vi "Initialize.vi"(8 "error in":errorcluster, 11 "Plugin in":refnum<class "StreamReader.lvclass">) -> (0 "error out":errorcluster, 3 "Plugin out":refnum<class "StreamReader.lvclass">)   [LabVIEW 2024, in "StreamReader.lvlib" / "StreamReader.lvclass"]
uses:
  StreamReader.lvclass
  C:/Program Files/National Instruments/LabVIEW 2024/vi.lib/FlexLogger/SDK/PluginSDK.lvlibp/PEFClasses/SDK/Plugin/Plugin.lvclass
  StreamReader Parameters.ctl
  <vilib>/FlexLogger/SDK/PluginSDK.lvlibp/PEFClasses/SDK/Processing Element/Timing Parameters.ctl
  <vilib>/FlexLogger/SDK/PluginSDK.lvlibp/PEFClasses/SDK/Processing Element/Timing Method.ctl
  StreamReader.lvclass/StreamReader.ctl
  StreamReader Strings.vi
  <vilib>/FlexLogger/SDK/PluginSDK.lvlibp/PEFClasses/SDK/Plugin/ParameterAccess/Write String.vi
  <vilib>/FlexLogger/SDK/PluginSDK.lvlibp/PEFClasses/SDK/Plugin/ParameterAccess/Write I32.vi
  <vilib>/FlexLogger/SDK/PluginSDK.lvlibp/PEFClasses/SDK/Plugin/Plugin.lvclass
  C:/Program Files/National Instruments/LabVIEW 2024/vi.lib/FlexLogger/SDK/PluginSDK.lvlibp/PEFClasses/SDK/Processing Element/Processing Element.lvclass
  C:/dev/niflexlogger-plugins/plugins/StreamReader/source/StreamReader/StreamReader.lvclass
  <vilib>/FlexLogger/SDK/PluginSDK.lvlibp/PEFClasses/SDK/Processing Element/Processing Element.lvclass
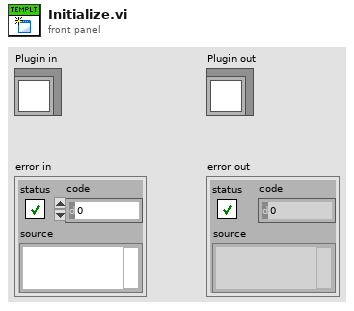
[diagram p1: front panel]
types:
  T1 = typedef "PluginSDK.lvlibp/Processing Element.lvclass/Timing Parameters.ctl" = cluster{"Timing Method":T2, "Timing Period (ms)":i32}
  T2 = typedef "PluginSDK.lvlibp/Processing Element.lvclass/Timing Method.ctl" = enum16{"Periodic", "Immediate", "On Data Ready", "Triggered"}
  T3 = typedef "StreamReader.lvlib/StreamReader.lvclass/StreamReader Parameters.ctl" = cluster{"Reader URL":string, "Writer URL":string, "Buffer Size":i32, "Reader endpoint":refnum<k21>, "Channel Names":string[]}
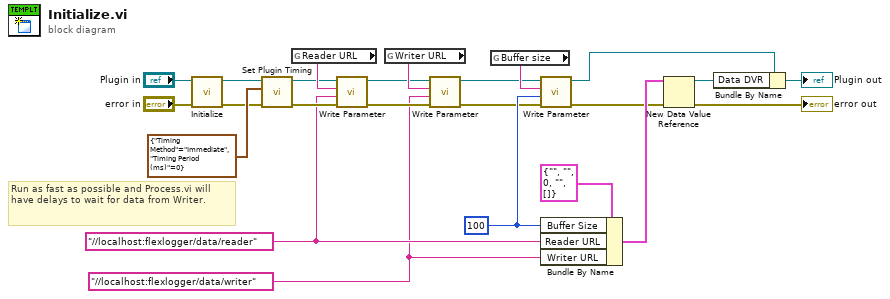
[diagram p0: block diagram]
diagram:
  w2 = "//localhost:flexlogger/data/reader" ("Value")
  w12 = 100 ("Value")
  w1 = "//localhost:flexlogger/data/writer" ("Value")
  # "Run as fast as possible and Process.vi will have delays to wait for data from Writer."
  n1 = call-parent "Initialize.vi"("error in (no error)"="error in", "Plugin in"="Plugin in") -> ("error out"=w6:errorcluster, "Plugin out"=w8:refnum<class "StreamReader.lvclass">)  [unwired: 8 in]
  n2 = call <vilib>:"Set Plugin Timing.vi"("error in (no error)"=w6, "Timing Parameters"=T1 {"Timing Method"=enum."Immediate", "Timing Period (ms)"=0}, "Plugin in"=w8) -> ("error out"=w5:errorcluster, "Plugin out"=w7:refnum<class "StreamReader.lvclass">)  [unwired: 7 in]
  n3 = global read "StreamReader Strings.vi" "Reader URL"() -> (w20:string)
  n4 = call-poly <vilib>:"Write Parameter.vi"("error in (no error)"=w5, "Value"=w2, "Name"=w20, "Plugin in"=w7) -> ("error out"=w18:errorcluster, "Plugin out"=w19:refnum<class "StreamReader.lvclass">)  [unwired: 6 in]
  n5 = global read "StreamReader Strings.vi" "Writer URL"() -> (w22:string)
  n6 = call-poly <vilib>:"Write Parameter.vi"("error in (no error)"=w18, "Value"=w1, "Name"=w22, "Plugin in"=w19) -> ("error out"=w3:errorcluster, "Plugin out"=w4:refnum<class "StreamReader.lvclass">)  [unwired: 6 in]
  n7 = global read "StreamReader Strings.vi" "Buffer size"() -> (w21:string)
  n8 = call-poly <vilib>:"Write Parameter.vi"("error in (no error)"=w3, "Value"=w12, "Name"=w21, "Plugin in"=w4) -> ("error out"=w11:errorcluster, "Plugin out"=w16:refnum<class "StreamReader.lvclass">)  [unwired: 6 in]
  n9 = Bundle By Name(cluster=T3 {"Reader URL"="", "Writer URL"="", "Buffer Size"=0, "Reader endpoint"="", "Channel Names"=[]} ("StreamReader Parameters"), "Buffer Size"=w12, "Reader URL"=w2, "Writer URL"=w1) -> (w13:T3)
  n10 = New Data Value Reference(data value=w13, error in=w11) -> (data value reference=w17:refnum<data-value>, error out=→"error out":errorcluster)
  n11 = Bundle By Name(cluster=w16, "Data DVR"=w17) -> (→"Plugin out":refnum<class "StreamReader.lvclass">)
